vi "Insert Into Array (Multi).vi"(8 "error in (no error)":errorcluster, 9 "index":i32, 10 "Array":refnum<class "JSON Datatype.lvclass">[](array[class]), 11 "JSON Array in":refnum<class "JSON Array.lvclass">) -> (0 "error out":errorcluster, 3 "JSON Array out":refnum<class "JSON Array.lvclass">)   [LabVIEW 2017, in "LVJSON.lvlib" / "JSON Array.lvclass"]
uses:
  JSON Array.lvclass
  JSON Datatype/JSON Datatype.lvclass
  JSON Array.lvclass/JSON Array.ctl
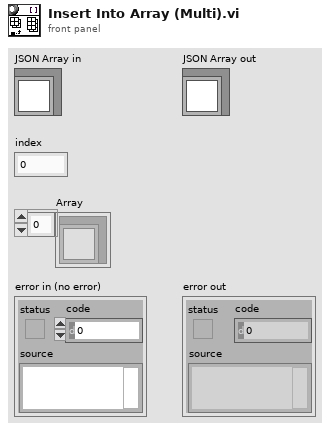
[diagram p1: front panel]
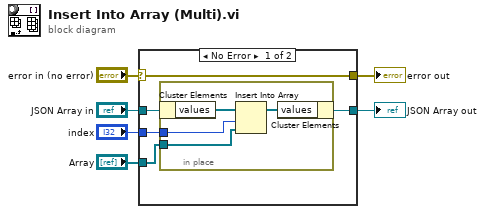
[diagram p0: block diagram]
diagram:
  n1 = case shown="No Error" "error in (no error)" {
    selector: "error in (no error)" -> [w7 w17]
    tunnel: [w7 w17] -> w5
    tunnel: [w8 w16] -> w3
    tunnel: "JSON Array in" -> [w9 w16]
    tunnel: "Array" -> [w10 _]
    tunnel: "index" -> [w11 _]
    frame No Error {
      n2 = in-place {
        in-place-border: w11 -> [w15]
        in-place-border: w10 -> [w14]
        n3 = in-place-cluster #1(w9) -> ("values"=w13:refnum<class "JSON Datatype.lvclass">[])
        n4 = Insert Into Array(array=w13, index=w15, new element=w14) -> (w12:refnum<class "JSON Datatype.lvclass">[])
        n5 = in-place-cluster #1("values"=w12) -> (w8:refnum<class "JSON Array.lvclass">)
      }
    }
    frame Error {
    }
  }
  "error out" <- w5
  "JSON Array out" <- w3
